vi "Update_with_correct_calib.vi"() -> ()   [LabVIEW 2010]
uses:
  Controls/File_Selector_Type.ctl
panel:
  in  "Previous Choice":path
  out "Files Processed":i32(slide) scale=0.0..1279.0
  out "Current Filename":path
  in  "Search String":string
  in  "At Dialog Prompt Add Metadata to:":T1
  in  "stop":bool
  out "Index":i32=22
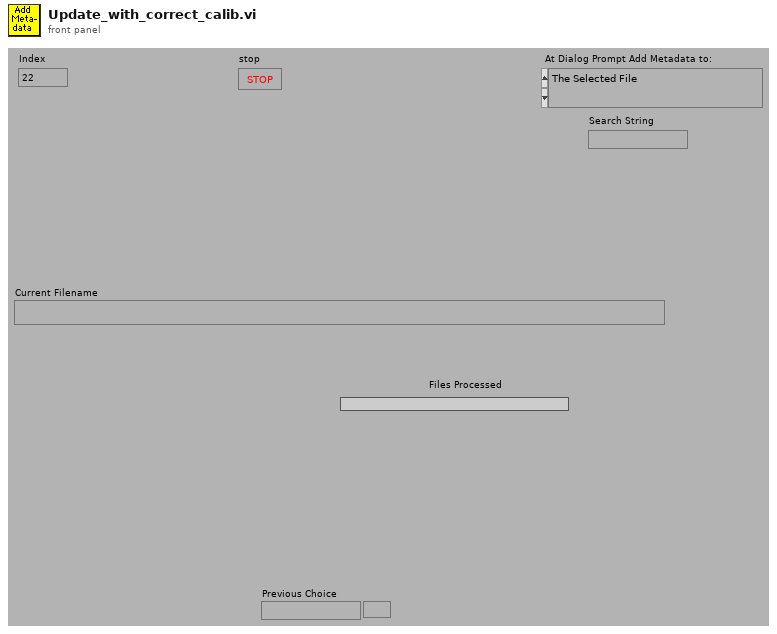
[diagram p1: front panel]
types:
  T1 = typedef "File_Selector_Type.ctl" = enum16{"The Selected File", "The Selected Folder", "Files containing the search string in the selected folder", "All files listed in selected file"}
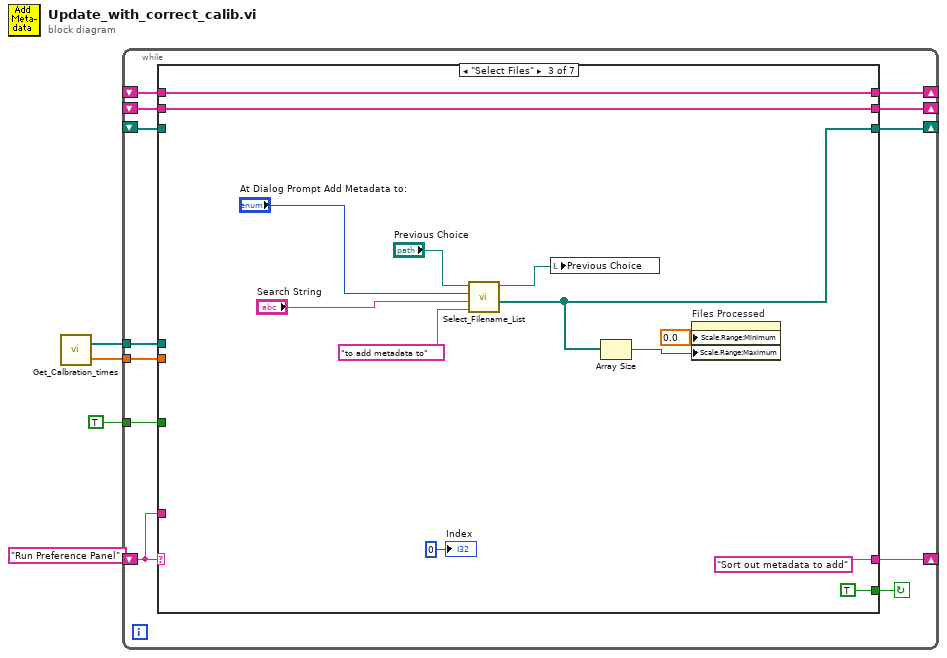
[diagram p0: block diagram]
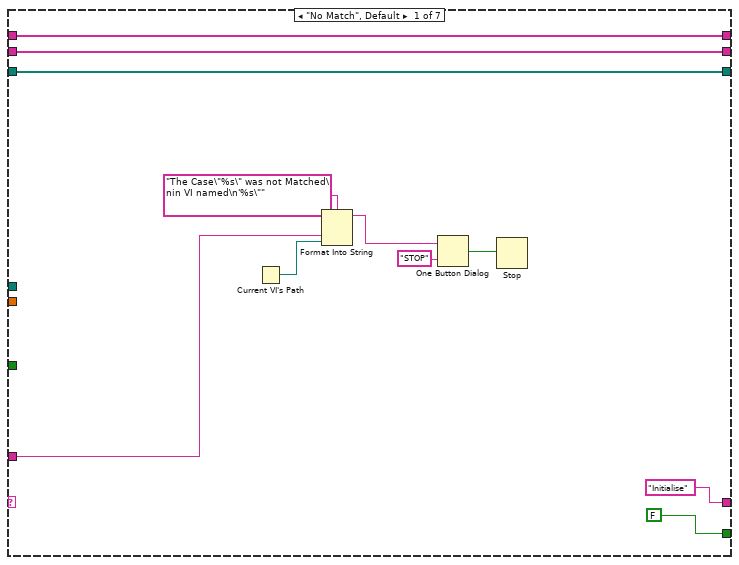
[diagram p2: hidden frame]
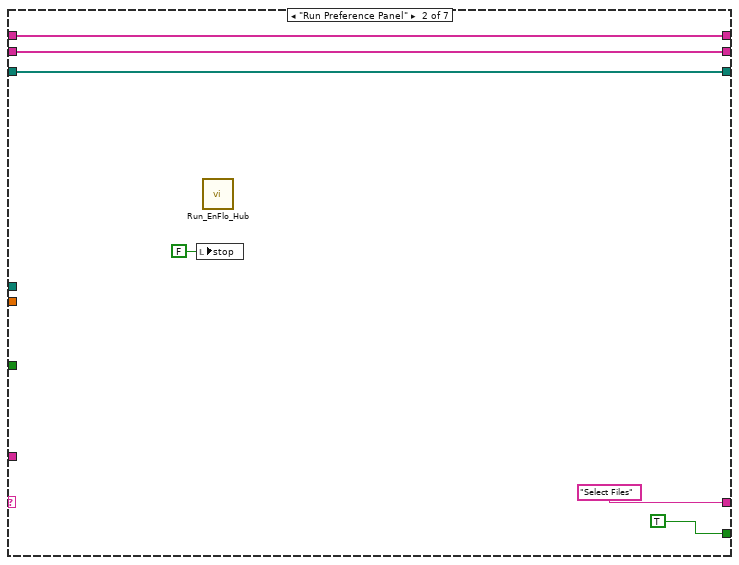
[diagram p3: hidden frame]
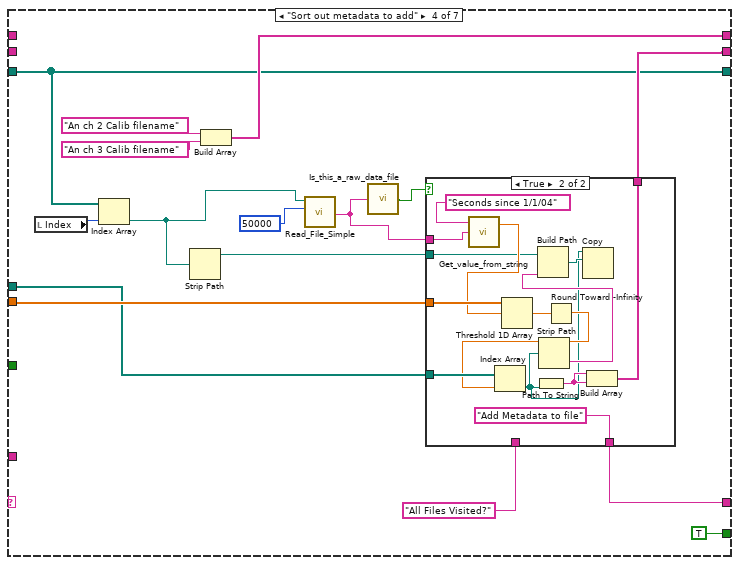
[diagram p4: hidden frame]
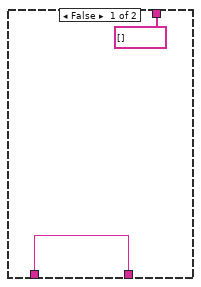
[diagram p5: hidden frame]
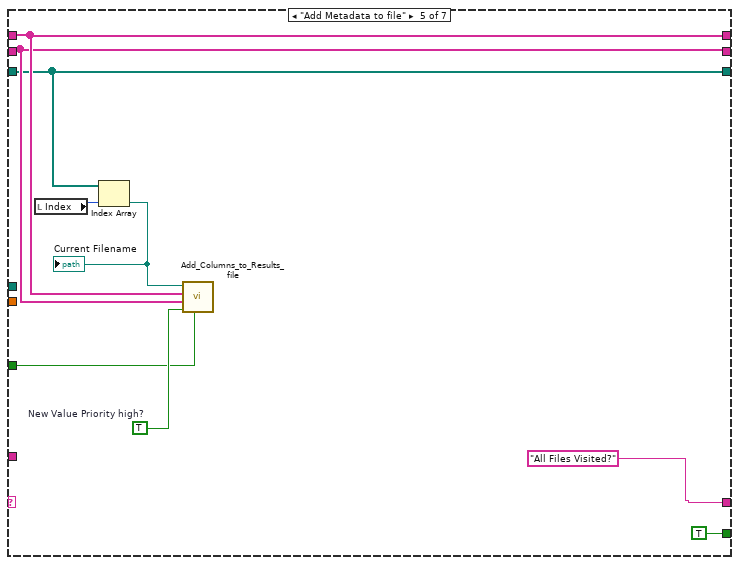
[diagram p6: hidden frame]
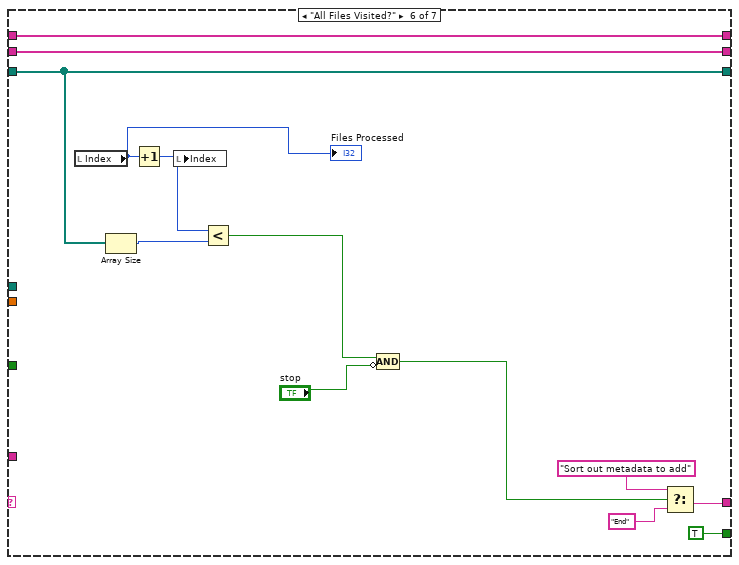
[diagram p7: hidden frame]
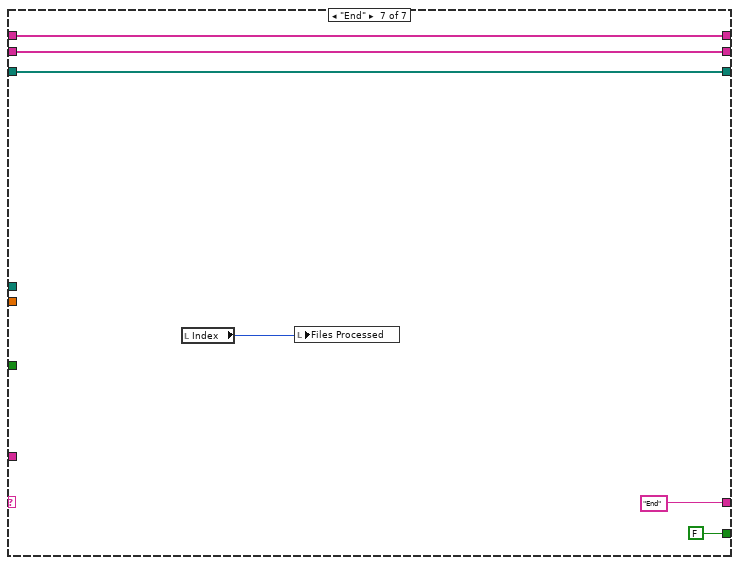
[diagram p8: hidden frame]
diagram:
  n1 = call "Get_Calbration_times.vi"() -> ("Seconds since 1904"=w3:dbl[], "Calib Filenames"=w2:path[])  [unwired: 2 in]
  n2 = while {
    tunnel: TRUE ("Edit Raw Data Header Info") -> [w7]
    shift-left: _ -> [w8]
    shift-right: [w9] -> _
    shift-left: _ -> [w11]
    shift-right: [w10] -> _
    shift-left: _ -> [w13]
    shift-right: [w14] -> _
    shift-left: "Run Preference Panel" -> [w15]
    shift-right: [w16] -> _
    tunnel: w3 -> [w6]
    tunnel: w2 -> [w5]
    stop <- w12 continue-if-true
    n3 = case shown="\"Select Files\"" w15 {
      tunnel: [FALSE TRUE TRUE TRUE TRUE TRUE FALSE] -> w12
      tunnel: ["Initialise" "Select Files" "Sort out metadata to add" w54 "All Files Visited?" w88 "End"] -> w16
      tunnel: w15 -> [w22 _ _ _ _ _ _]
      tunnel: [w19 w32 w38 w52 w80 w100 w103] -> w14
      tunnel: w13 -> [w19 w32 _ w52 w80 w100 w103]
      tunnel: w11 -> [w18 w30 w41 _ w83 w95 w106]
      tunnel: [w18 w30 w41 w57 w83 w95 w106] -> w10
      tunnel: [w17 w29 w45 w55 w82 w94 w105] -> w9
      tunnel: w8 -> [w17 w29 w45 _ w82 w94 w105]
      tunnel: w7 -> [_ _ _ _ w81 _ _]
      tunnel: w6 -> [_ _ _ w60 _ _ _]
      tunnel: w5 -> [_ _ _ w56 _ _ _]
      frame "No Match", Default {
        n4 = Current VI's Path() -> (path=w21:path)
        n5 = Format Into String(format string="The Case\"%s\" was not Matched\nin VI named\n'%s\"" ("Format String"), w22, w21) -> (resulting string=w25:string)  [unwired: 2 in, 1 out]
        n6 = One Button Dialog(message=w25, button name ("OK")="STOP") -> (true=w23:bool)
        n7 = Stop(stop? (T)=w23) -> ()
      }
      frame "Run Preference Panel" {
        n8 = local write "stop"(FALSE ("stop")) -> ()
        n9 = call "Run_EnFlo_Hub.vi"() -> ()  [unwired: 8 in]
      }
      frame "Select Files" {
        n10 = call "Select_Filename_List.vi"("File Type"="to add metadata to", "Search String"="Search String", "At Dialog Prompt Post Process"="At Dialog Prompt Add Metadata to:", "Previous Choice"="Previous Choice") -> ("Selected files"=w38:path[], "Choosen path"=w35:path)  [unwired: 2 in, 1 out]
        n11 = local write "Previous Choice"(w35) -> ()
        n12 = Array Size(array=w38) -> (size(s)=w37:i32)
        n13 = property on="Files Processed" class="Slide (strict)"("Scale.Range:Minimum"=0.0, "Scale.Range:Maximum"=w37) -> ()  [unwired: 2 in, 2 out]
        "Index" <- 0 ("Index")
      }
      frame "Sort out metadata to add" {
        n14 = local read "Index"() -> (w61:i32)
        n15 = Index Array(array=w52, index=w61) -> (element=w51:path)
        n16 = Strip Path(path=w51) -> (stripped path=w50:path)  [unwired: 1 out]
        n17 = Build Array("An ch 2 Calib filename", "An ch 3 Calib filename") -> (w57:string[])
        n18 = call "Read_File_Simple.vi"("Filename"=w51, "number of characters (all:-1)"=50000) -> ("string"=w48:string)  [unwired: 3 in, 5 out]
        n19 = call "Is_this_a_raw_data_file.vi"("character string"=w48) -> ("Raw Dat File?"=w49:bool)  [unwired: 2 in]
        n20 = case shown="True" w49 {
          tunnel: w48 -> [_ w77]
          tunnel: w60 -> [_ w76]
          tunnel: w56 -> [_ w73]
          tunnel: [string[] [] w70] -> w55
          tunnel: [w63 "Add Metadata to file"] -> w54
          tunnel: "All Files Visited?" -> [w63 _]
          tunnel: w50 -> [_ w66]
          frame False {
          }
          frame True {
            n21 = call "Get_value_from_string.vi"("Input string"=w77, "Variable name"="Seconds since 1/1/04") -> ("Value"=w75:dbl)  [unwired: 1 in, 1 out]
            n22 = Threshold 1D Array(2:w75, 3:w76) -> (0:w74:dbl)  [unwired: 1 in]
            n23 = Round Toward -Infinity(1:w74) -> (0:w72:dbl)
            n24 = Index Array(array=w73, index=w72) -> (element=w65:path)
            n25 = Path To String(path=w65) -> (string=w71:string)
            n26 = Strip Path(path=w65) -> (name=w67:string)  [unwired: 1 out]
            n27 = Build Path(base path=w66, name or relative path=w67) -> (appended path=w68:path)
            n28 = Copy(10:w68, 11:w65) -> ()  [unwired: 3 in, 3 out]
            n29 = Build Array(w71, w71) -> (w70:string[])
          }
        }
      }
      frame "Add Metadata to file" {
        w84 = TRUE  # New Value Priority high?
        n30 = local read "Index"() -> (w85:i32)
        n31 = Index Array(array=w80, index=w85) -> (element=w86:path)
        "Current Filename" <- w86
        n32 = call "Add_Columns_to_Results_file.vi"("Edit Raw Data Header Info"=w81, "New Value Priority high?"=w84, "New Values In"=w82, "New Chs In"=w83, "Data filename"=w86) -> ()  [unwired: 5 out]
      }
      frame "All Files Visited?" {
        n33 = local read "Index"() -> (w93:i32)
        "Files Processed" <- w93
        n34 = Array Size(array=w100) -> (size(s)=w98:i32)
        n35 = Increment(x=w93) -> (x+1=w99:i32)
        n36 = local write "Index"(w99) -> ()
        n37 = Less?(x=w99, y=w98) -> (x < y?=w96:bool)
        n38 = Compound Arithmetic op=AND(w96, invert "stop") -> (w91:bool)
        n39 = Select(t="Sort out metadata to add", s=w91, f="End") -> (s? t:f=w88:string)
      }
      frame "End" {
        n40 = local read "Index"() -> (w101:i32)
        n41 = local write "Files Processed"(w101) -> ()
      }
    }
  }
